vi "set_ellipsoid.vi"(8 "error in (no error)":errorcluster, 10 "ellipsoid parameter cluster":T1={"a"=0.0, "b"=0.125, "c"=0.5, "d"=0.015625, "e"=0.5, "k"=0, "width"=0.0} {"a" format="%.16g"; "b" format="%.16g"; "c" format="%.16g"; "d" format="%.16g"}, 11 "FPGAWrapperMH120124RAPS_PXI7813R in":refnum<class "FPGAWrapperMH120124RAPS_PXI7813R.lvclass">) -> (0 "error out":errorcluster, 3 "FPGAWrapperMH120124RAPS_PXI7813R out":refnum<class "FPGAWrapperMH120124RAPS_PXI7813R.lvclass">)   [LabVIEW 2010, in "FPGAWrapperMH120124RAPS_PXI7813R.lvclass"]
uses:
  FPGAWrapperMH120124RAPS_PXI7813R.lvclass
  fpgaVIsAndControls/ellipsoid_parameters_cluster.ctl
  FPGAWrapperMH120124RAPS_PXI7813R.lvclass/FPGAWrapperMH120124RAPS_PXI7813R.ctl
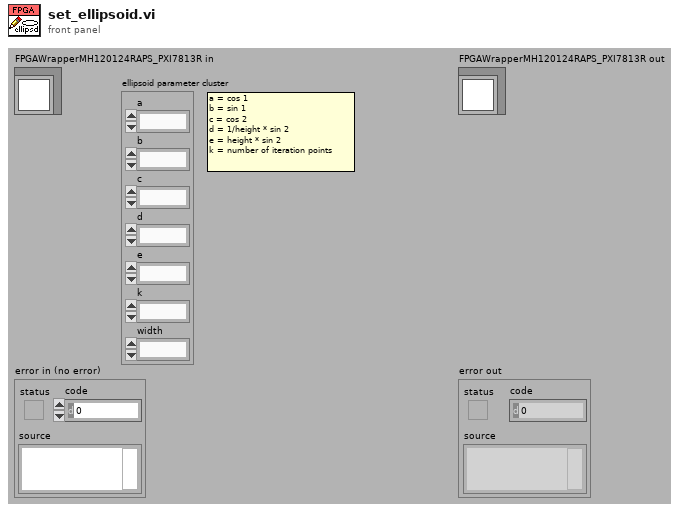
[diagram p1: front panel]
types:
  T1 = typedef "ellipsoid_parameters_cluster.ctl" = cluster{"a":fxp<+/-,16,1>, "b":fxp<+/-,16,1>, "c":fxp<+/-,16,1>, "d":fxp<+/-,16,1>, "e":fxp<+/-,24,16>, "k":u16, "width":fxp<+,16,16>}
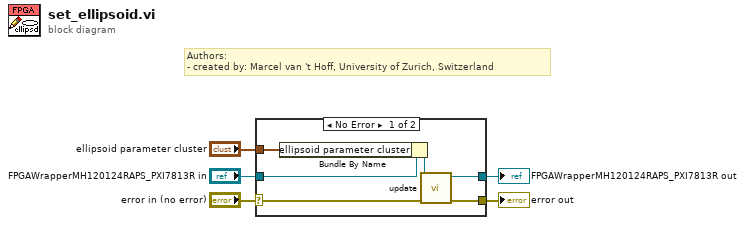
[diagram p0: block diagram]
diagram:
  # "Authors: \n- created by: Marcel van 't Hoff, University of Zurich, Switzerland"
  n1 = case shown="No Error" "error in (no error)" {
    selector: "error in (no error)" -> [w7 w13]
    tunnel: [w6 w13] -> w4
    tunnel: [w8 w12] -> w2
    tunnel: "FPGAWrapperMH120124RAPS_PXI7813R in" -> [w11 w12]
    tunnel: "ellipsoid parameter cluster" -> [w10 _]
    frame No Error {
      n2 = Bundle By Name(cluster=w11, "ellipsoid parameter cluster"=w10) -> (w9:refnum<class "FPGAWrapperMH120124RAPS_PXI7813R.lvclass">)
      n3 = call-dynamic "update.vi"("error in (no error)"=w7, "FPGAWrapperMH120124RAPS_PXI7813R in"=w9) -> ("error out"=w6:errorcluster, "FPGAWrapperMH120124RAPS_PXI7813R out"=w8:refnum<class "FPGAWrapperMH120124RAPS_PXI7813R.lvclass">)  [unwired: 8 in]
    }
    frame Error {
    }
  }
  "error out" <- w4
  "FPGAWrapperMH120124RAPS_PXI7813R out" <- w2
